vi "WT CONFIG.vi"(7 "WT 1600?":bool, 8 "error in (no error)":errorcluster, 10 "WT1600 Config ing 2":T1={"Wiring A (0: 1P2W)"=0, "Wiring B (0: 1P2W)"=0, "Wiring C (0: 1P2W)"=0, "V Range (12: 1000)"=12, "V Element (0: All)"=0, "A Element (0: All)"=0, "A Range (9: 5A)"=9, "A Sensor Ratio(mV/A) (10.0000) "=10.0, "Zero Cross Filter (0: OFF)"=0, "Line Filter (0: OFF)"=0, "PT Ratio (1.0000)"=1.0, "Scaling (F: OFF)"=FALSE, "CT Ratio (1.0000)"=1.0, "Scaling Factor (1.0000)"=1.0, "Filter Element (0: All)"=0, "Display Format (0: Numeric)"=0, "Normal Item Amount (1: 4)"=1, "Harmonics Item Amount (1: 4)"=1, "Average Type (0: OFF)"=0, "Average Count (2: 8)"=2, "A Range (9: 5A) 2"=9, "A Sensor Ratio(mV/A) (10.0000)  2"=10.0, "Zero Cross Filter (0: OFF) 2"=0, "Line Filter (0: OFF) 2"=0, "PT Ratio (1.0000) 2"=1.0, "Scaling (F: OFF) 2"=FALSE, "CT Ratio (1.0000) 2"=1.0, "Scaling Factor (1.0000) 2"=1.0, "CUT OFF FREQ"=0.0} {"Scaling Factor (1.0000) 2" min=0.0001 max=99999.9999 step=0.0001 format="%.4f"; "CT Ratio (1.0000) 2" min=0.0001 max=99999.9999 step=0.0001 format="%.4f"; "PT Ratio (1.0000) 2" min=0.0001 max=99999.9999 step=0.0001 format="%.4f"; "Line Filter (0: OFF) 2" items=["OFF", "500Hz", "5.5kHz"]; "Zero Cross Filter (0: OFF) 2" items=["OFF", "500Hz"]; "A Sensor Ratio(mV/A) (10.0000)  2" min=0.0001 max=99999.9999 step=0.0001 format="%.4f"; "A Range (9: 5A) 2" items=["AUTO", "10 mA", "20 mA", "50 mA", "100 mA", "200 mA", "500 mA", "1 A", "2 A", "5 A", "10 A", "20 A", "50 A", "S-AUTO", "50 mV", "100 mV", "250 mV", "500 mV", "1 V", "2.5 V", "5 V", "10 V"]; "Average Count (2: 8)" items=["2", "4", "8", "16", "32", "64", "128", "256"]; "Average Type (0: OFF)" items=["OFF", "Linear", "Exponent"]; "Harmonics Item Amount (1: 4)" items=["-", "4", "8", "16", "Single List", "Dual List", "Sigma List"]; "Normal Item Amount (1: 4)" items=["ALL", "4", "8", "16", "42", "78"]; "Display Format (0: Numeric)" items=["Numeric", "Wave", "Bar", "Vector", "Trend", "Numeric & Wave", "Numeric & Bar", "Numeric & Trend", "Wave & Bar", "Wave & Trend", "Bar & Trend", "Information"]; "Filter Element (0: All)" items=["All", "Element 1", "Element 2", "Element 3", "Element 4", "Element 5", "Element 6"]; "Scaling Factor (1.0000)" min=0.0001 max=99999.9999 step=0.0001 format="%.4f"; "CT Ratio (1.0000)" min=0.0001 max=99999.9999 step=0.0001 format="%.4f"; "PT Ratio (1.0000)" min=0.0001 max=99999.9999 step=0.0001 format="%.4f"; "Line Filter (0: OFF)" items=["OFF", "500Hz", "5.5kHz"]; "Zero Cross Filter (0: OFF)" items=["OFF", "500Hz"]; "A Sensor Ratio(mV/A) (10.0000)" min=0.0001 max=99999.9999 step=0.0001 format="%.4f"; "A Range (9: 5A)" items=["AUTO", "10 mA", "20 mA", "50 mA", "100 mA", "200 mA", "500 mA", "1 A", "2 A", "5 A", "10 A", "20 A", "50 A", "S-AUTO", "50 mV", "100 mV", "250 mV", "500 mV", "1 V", "2.5 V", "5 V", "10 V"]; "A Element (0: All)" items=["All", "Element 1", "Element 2", "Element 3", "Element 4", "Element 5", "Element 6"]; "V Element (0: All)" items=["All", "Element 1", "Element 2", "Element 3", "Element 4", "Element 5", "Element 6"]; "V Range (12: 1000)" items=["AUTO", "1.5", "3", "6", "10", "15", "30", "60", "100", "150", "300", "600", "1000"]; "Wiring C (0: 1P2W)" items=["1P2W", "1P3W", "3P3W", "3P4W", "3V3A", "NONE"]; "Wiring B (0: 1P2W)" items=["1P2W", "1P3W", "3P3W", "3P4W", "3V3A", "NONE"]; "Wiring A (0: 1P2W)" items=["1P2W", "1P3W", "3P3W", "3P4W", "3V3A"]}, 11 "VISA Refnum in":refnum<visa-resource-name>) -> (0 "error OUT":errorcluster, 3 "VISA OUT":refnum<visa-resource-name>)   [LabVIEW 2019]
panel:
  # "ON\nOFF"
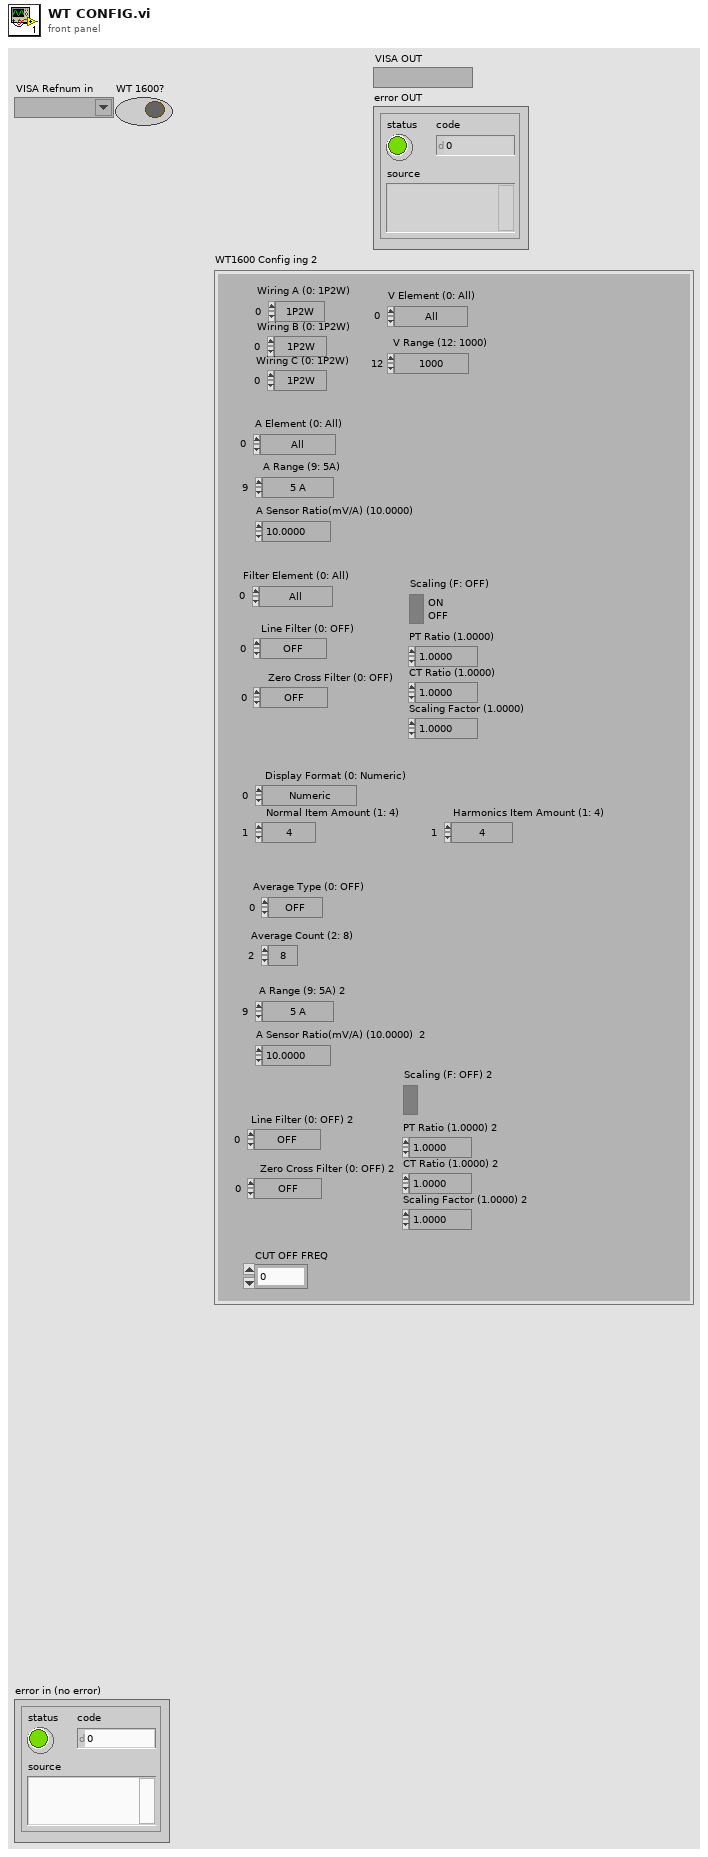
[diagram p1: front panel]
types:
  T1 = cluster{"Wiring A (0: 1P2W)":u16, "Wiring B (0: 1P2W)":u16, "Wiring C (0: 1P2W)":u16, "V Range (12: 1000)":u16, "V Element (0: All)":u16, "A Element (0: All)":u16, "A Range (9: 5A)":u16, "A Sensor Ratio(mV/A) (10.0000) ":dbl, "Zero Cross Filter (0: OFF)":u16, "Line Filter (0: OFF)":u16, "PT Ratio (1.0000)":dbl, "Scaling (F: OFF)":bool, "CT Ratio (1.0000)":dbl, "Scaling Factor (1.0000)":dbl, "Filter Element (0: All)":u16, "Display Format (0: Numeric)":u16, "Normal Item Amount (1: 4)":u16, "Harmonics Item Amount (1: 4)":u16, "Average Type (0: OFF)":u16, "Average Count (2: 8)":u16, "A Range (9: 5A) 2":u16, "A Sensor Ratio(mV/A) (10.0000)  2":dbl, "Zero Cross Filter (0: OFF) 2":u16, "Line Filter (0: OFF) 2":u16, "PT Ratio (1.0000) 2":dbl, "Scaling (F: OFF) 2":bool, "CT Ratio (1.0000) 2":dbl, "Scaling Factor (1.0000) 2":dbl, "CUT OFF FREQ":dbl}
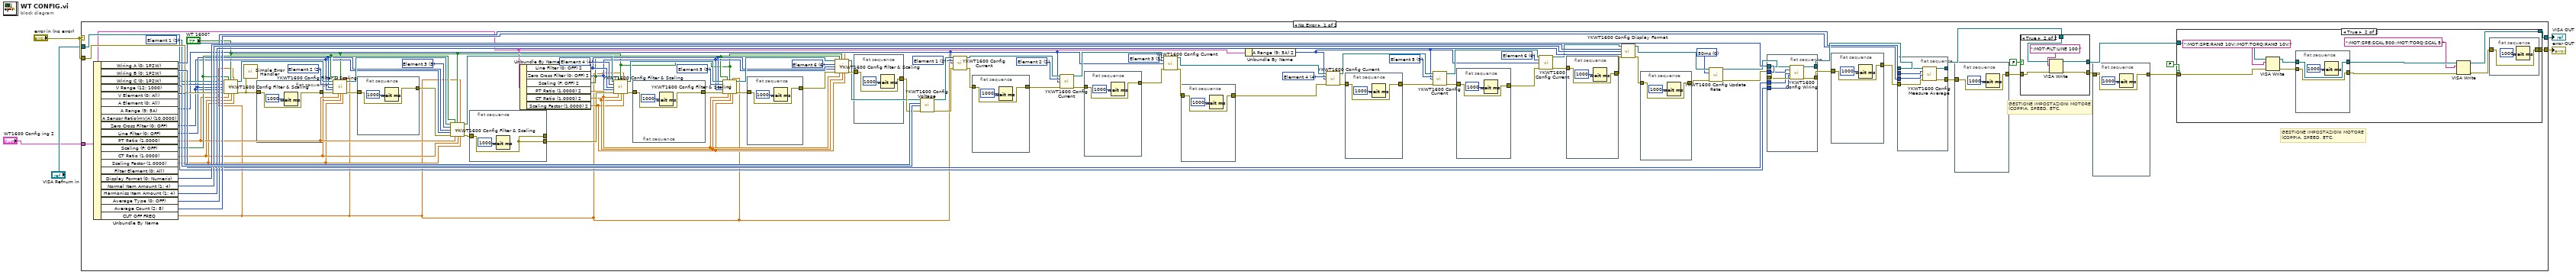
[diagram p0: block diagram]
diagram:
  n1 = case shown="No Error" "error in (no error)" {
    tunnel: "WT1600 Config ing 2" -> [w13 _]
    tunnel: "error in (no error)" -> [w76 w175]
    tunnel: "VISA Refnum in" -> [w75 w174]
    tunnel: [w74 w174] -> w3
    tunnel: [w73 w175] -> w2
    frame No Error {
      w26 = u16 6 items=["All", "Element 1", "Element 2", "Element 3", "Element 4", "Element 5", "Element 6"] ("Element (0: All)")
      w25 = u16 5 items=["All", "Element 1", "Element 2", "Element 3", "Element 4", "Element 5", "Element 6"] ("Element (0: All)")
      w24 = u16 4 items=["All", "Element 1", "Element 2", "Element 3", "Element 4", "Element 5", "Element 6"] ("Element (0: All)")
      w22 = u16 3 items=["All", "Element 1", "Element 2", "Element 3", "Element 4", "Element 5", "Element 6"] ("Element (0: All)")
      w23 = u16 2 items=["All", "Element 1", "Element 2", "Element 3", "Element 4", "Element 5", "Element 6"] ("Element (0: All)")
      w21 = u16 1 items=["All", "Element 1", "Element 2", "Element 3", "Element 4", "Element 5", "Element 6"] ("Element (0: All)")
      w52 = u16 6 items=["All", "Element 1", "Element 2", "Element 3", "Element 4", "Element 5", "Element 6"] ("Element (0: All)")
      w53 = u16 5 items=["All", "Element 1", "Element 2", "Element 3", "Element 4", "Element 5", "Element 6"] ("Element (0: All)")
      w54 = u16 4 items=["All", "Element 1", "Element 2", "Element 3", "Element 4", "Element 5", "Element 6"] ("Element (0: All)")
      w55 = u16 3 items=["All", "Element 1", "Element 2", "Element 3", "Element 4", "Element 5", "Element 6"] ("Element (0: All)")
      w51 = u16 2 items=["All", "Element 1", "Element 2", "Element 3", "Element 4", "Element 5", "Element 6"] ("Element (0: All)")
      w56 = u16 1 items=["All", "Element 1", "Element 2", "Element 3", "Element 4", "Element 5", "Element 6"] ("Element (0: All)")
      w82 = u16 0 items=["50ms", "100ms", "200ms", "500ms", "1s", "2s", "5s"] ("Update Rate (3: 500ms)")
      # "GESTIONE IMPOSTAZIONI MOTORE\n(COPPIA, SPEED, ETC."
      # "GESTIONE IMPOSTAZIONI MOTORE\n(COPPIA, SPEED, ETC."
      n2 = Unbundle By Name(w13) -> ("Wiring A (0: 1P2W)"=w93:u16, "Wiring B (0: 1P2W)"=w92:u16, "Wiring C (0: 1P2W)"=w91:u16, "V Range (12: 1000)"=w101:u16, "V Element (0: All)"=w100:u16, "A Range (9: 5A)"=w20:u16, "Zero Cross Filter (0: OFF)"=w48:u16, "Line Filter (0: OFF)"=w49:u16, "PT Ratio (1.0000)"=w47:dbl, "Scaling (F: OFF)"=w50:bool, "CT Ratio (1.0000)"=w46:dbl, "Scaling Factor (1.0000)"=w45:dbl, "Display Format (0: Numeric)"=w99:u16, "Normal Item Amount (1: 4)"=w98:u16, "Harmonics Item Amount (1: 4)"=w97:u16, "Average Type (0: OFF)"=w95:u16, "Average Count (2: 8)"=w94:u16, "CUT OFF FREQ"=w6:dbl)  [unwired: 3 out]
      n3 = call "YKWT1600 Config Filter & Scaling.vi"("VISA session"=w75, "Scaling (F: OFF)"=w50, "WT 1600?"="WT 1600?", "Cutoff Frequency (0.5 kHz)"=w6, "Element (0: All)"=w56, "Line Filter (0: OFF)"=w49, "WT 1600 Zero Cross Filter (0: OFF)"=w48, "error in (no error)"=w76, "PT Ratio (1.0000)"=w47, "CT Ratio (1.0000)"=w46, "Scaling Factor (1.0000)"=w45) -> ("dup VISA session"=w72:refnum<visa-resource-name>, "error out"=w10:errorcluster)  [unwired: 3 out]
      n4 = call <vilib>:"Simple Error Handler.vi"("error in (no error)"=w10) -> ()  [unwired: 4 in, 5 out]
      n5 = flat-sequence {
        tunnel: w10 -> [w165]
        tunnel: [w165] -> w9
        frame #0 {
          n6 = Wait (ms)(milliseconds to wait=1000) -> ()  [unwired: 1 out]
        }
      }
      n7 = call "YKWT1600 Config Filter & Scaling.vi"("VISA session"=w72, "Scaling (F: OFF)"=w50, "WT 1600?"="WT 1600?", "Cutoff Frequency (0.5 kHz)"=w6, "Element (0: All)"=w51, "Line Filter (0: OFF)"=w49, "WT 1600 Zero Cross Filter (0: OFF)"=w48, "error in (no error)"=w9, "PT Ratio (1.0000)"=w47, "CT Ratio (1.0000)"=w46, "Scaling Factor (1.0000)"=w45) -> ("dup VISA session"=w58:refnum<visa-resource-name>, "error out"=w71:errorcluster)  [unwired: 3 out]
      n8 = flat-sequence {
        tunnel: w71 -> [w163]
        tunnel: [w163] -> w70
        frame #0 {
          n9 = Wait (ms)(milliseconds to wait=1000) -> ()  [unwired: 1 out]
        }
      }
      n10 = call "YKWT1600 Config Filter & Scaling.vi"("VISA session"=w58, "Scaling (F: OFF)"=w50, "WT 1600?"="WT 1600?", "Cutoff Frequency (0.5 kHz)"=w6, "Element (0: All)"=w55, "Line Filter (0: OFF)"=w49, "WT 1600 Zero Cross Filter (0: OFF)"=w48, "error in (no error)"=w70, "PT Ratio (1.0000)"=w47, "CT Ratio (1.0000)"=w46, "Scaling Factor (1.0000)"=w45) -> ("dup VISA session"=w61:refnum<visa-resource-name>, "error out"=w69:errorcluster)  [unwired: 3 out]
      n11 = flat-sequence {
        tunnel: [w160] -> _
        tunnel: [w160] -> w68
        tunnel: w69 -> [w160]
        frame #0 {
          n12 = Wait (ms)(milliseconds to wait=1000) -> ()  [unwired: 1 out]
        }
      }
      n13 = Unbundle By Name(w13) -> ("Line Filter (0: OFF) 2"=w19:u16, "Zero Cross Filter (0: OFF) 2"=w18:u16, "Scaling (F: OFF) 2"=w17:bool, "PT Ratio (1.0000) 2"=w16:dbl, "CT Ratio (1.0000) 2"=w15:dbl, "Scaling Factor (1.0000) 2"=w14:dbl)
      n14 = call "YKWT1600 Config Filter & Scaling.vi"("VISA session"=w61, "Scaling (F: OFF)"=w17, "WT 1600?"="WT 1600?", "Cutoff Frequency (0.5 kHz)"=w6, "Element (0: All)"=w54, "Line Filter (0: OFF)"=w19, "WT 1600 Zero Cross Filter (0: OFF)"=w18, "error in (no error)"=w68, "PT Ratio (1.0000)"=w16, "CT Ratio (1.0000)"=w15, "Scaling Factor (1.0000)"=w14) -> ("dup VISA session"=w60:refnum<visa-resource-name>, "error out"=w67:errorcluster)  [unwired: 3 out]
      n15 = flat-sequence {
        tunnel: w67 -> [w159]
        tunnel: [w159] -> w66
        frame #0 {
          n16 = Wait (ms)(milliseconds to wait=1000) -> ()  [unwired: 1 out]
        }
      }
      n17 = call "YKWT1600 Config Filter & Scaling.vi"("VISA session"=w60, "Scaling (F: OFF)"=w17, "WT 1600?"="WT 1600?", "Cutoff Frequency (0.5 kHz)"=w6, "Element (0: All)"=w53, "Line Filter (0: OFF)"=w19, "WT 1600 Zero Cross Filter (0: OFF)"=w18, "error in (no error)"=w66, "PT Ratio (1.0000)"=w16, "CT Ratio (1.0000)"=w15, "Scaling Factor (1.0000)"=w14) -> ("dup VISA session"=w59:refnum<visa-resource-name>, "error out"=w65:errorcluster)  [unwired: 3 out]
      n18 = flat-sequence {
        tunnel: w65 -> [w157]
        tunnel: [w157] -> w64
        frame #0 {
          n19 = Wait (ms)(milliseconds to wait=1000) -> ()  [unwired: 1 out]
        }
      }
      n20 = call "YKWT1600 Config Filter & Scaling.vi"("VISA session"=w59, "Scaling (F: OFF)"=w17, "WT 1600?"="WT 1600?", "Cutoff Frequency (0.5 kHz)"=w6, "Element (0: All)"=w52, "Line Filter (0: OFF)"=w19, "WT 1600 Zero Cross Filter (0: OFF)"=w18, "error in (no error)"=w64, "PT Ratio (1.0000)"=w16, "CT Ratio (1.0000)"=w15, "Scaling Factor (1.0000)"=w14) -> ("dup VISA session"=w57:refnum<visa-resource-name>, "error out"=w63:errorcluster)  [unwired: 3 out]
      n21 = flat-sequence {
        tunnel: w63 -> [w155]
        tunnel: [w155] -> w62
        frame #0 {
          n22 = Wait (ms)(milliseconds to wait=1000) -> ()  [unwired: 1 out]
        }
      }
      n23 = call "YKWT1600 Config Voltage.vi"("VISA session"=w57, "Element (0: All)"=w100, "V Range (12: 1000)"=w101, "error in (no error)"=w62) -> ("dup VISA session"=w103:refnum<visa-resource-name>, "error out"=w102:errorcluster)  [unwired: 10 out]
      n24 = call "YKWT1600 Config Current.vi"("VISA session"=w103, "Element (0: All)"=w21, "A Range (9: 5A)"=w20, "error in (no error)"=w102) -> ("dup VISA session"=w28:refnum<visa-resource-name>, "error out"=w34:errorcluster)  [unwired: 1 in, 9 out]
      n25 = flat-sequence {
        tunnel: w34 -> [w153]
        tunnel: [w153] -> w44
        frame #0 {
          n26 = Wait (ms)(milliseconds to wait=1000) -> ()  [unwired: 1 out]
        }
      }
      n27 = call "YKWT1600 Config Current.vi"("VISA session"=w28, "Element (0: All)"=w23, "A Range (9: 5A)"=w20, "error in (no error)"=w44) -> ("dup VISA session"=w32:refnum<visa-resource-name>, "error out"=w43:errorcluster)  [unwired: 1 in, 9 out]
      n28 = flat-sequence {
        tunnel: w43 -> [w151]
        tunnel: [w151] -> w42
        frame #0 {
          n29 = Wait (ms)(milliseconds to wait=1000) -> ()  [unwired: 1 out]
        }
      }
      n30 = call "YKWT1600 Config Current.vi"("VISA session"=w32, "Element (0: All)"=w22, "A Range (9: 5A)"=w20, "error in (no error)"=w42) -> ("dup VISA session"=w31:refnum<visa-resource-name>, "error out"=w41:errorcluster)  [unwired: 1 in, 9 out]
      n31 = flat-sequence {
        tunnel: w41 -> [w149]
        tunnel: [w149] -> w40
        frame #0 {
          n32 = Wait (ms)(milliseconds to wait=1000) -> ()  [unwired: 1 out]
        }
      }
      n33 = Unbundle By Name(w13) -> ("A Range (9: 5A) 2"=w12:u16)
      n34 = call "YKWT1600 Config Current.vi"("VISA session"=w31, "Element (0: All)"=w24, "A Range (9: 5A)"=w12, "error in (no error)"=w40) -> ("dup VISA session"=w30:refnum<visa-resource-name>, "error out"=w39:errorcluster)  [unwired: 1 in, 9 out]
      n35 = flat-sequence {
        tunnel: w39 -> [w147]
        tunnel: [w147] -> w38
        frame #0 {
          n36 = Wait (ms)(milliseconds to wait=1000) -> ()  [unwired: 1 out]
        }
      }
      n37 = call "YKWT1600 Config Current.vi"("VISA session"=w30, "Element (0: All)"=w25, "A Range (9: 5A)"=w12, "error in (no error)"=w38) -> ("dup VISA session"=w29:refnum<visa-resource-name>, "error out"=w37:errorcluster)  [unwired: 1 in, 9 out]
      n38 = flat-sequence {
        tunnel: [w144] -> w36
        tunnel: w37 -> [w144]
        frame #0 {
          n39 = Wait (ms)(milliseconds to wait=1000) -> ()  [unwired: 1 out]
        }
      }
      n40 = call "YKWT1600 Config Current.vi"("VISA session"=w29, "Element (0: All)"=w26, "A Range (9: 5A)"=w12, "error in (no error)"=w36) -> ("dup VISA session"=w27:refnum<visa-resource-name>, "error out"=w35:errorcluster)  [unwired: 1 in, 9 out]
      n41 = flat-sequence {
        tunnel: [w142] -> w33
        tunnel: w35 -> [w142]
        frame #0 {
          n42 = Wait (ms)(milliseconds to wait=1000) -> ()  [unwired: 1 out]
        }
      }
      n43 = call "YKWT1600 Config Display Format.vi"("VISA session"=w27, "Display Format (0: Numeric)"=w99, "Normal Item Amount (1: 4)"=w98, "Harmonics Item Amount (1: 4)"=w97, "error in (no error)"=w33) -> ("dup VISA session"=w86:refnum<visa-resource-name>, "error out"=w87:errorcluster)  [unwired: 9 out]
      n44 = flat-sequence {
        tunnel: w87 -> [w171]
        tunnel: [w171] -> w84
        frame #0 {
          n45 = Wait (ms)(milliseconds to wait=1000) -> ()  [unwired: 1 out]
        }
      }
      n46 = call "YKWT1600 Config Update Rate.vi"("VISA session"=w86, "Update Rate (3: 500ms)"=w82, "error in (no error)"=w84) -> ("dup VISA session"=w85:refnum<visa-resource-name>, "error out"=w83:errorcluster)  [unwired: 11 in]
      n47 = flat-sequence {
        tunnel: [w134] -> w96
        tunnel: [w135] -> w78
        tunnel: w85 -> [w133]
        tunnel: w83 -> [w132]
        tunnel: w91 -> [w129]
        tunnel: w92 -> [w130]
        tunnel: w93 -> [w131]
        frame #0 {
          n48 = call "YKWT1600 Config Wiring.vi"("VISA session"=w133, "Wiring A (0: 1P2W)"=w131, "Wiring B (0: 1P2W)"=w130, "Wiring C (0: 1P2W)"=w129, "error in (no error)"=w132) -> ("dup VISA session"=w134:refnum<visa-resource-name>, "error out"=w135:errorcluster)  [unwired: 9 out]
        }
      }
      n49 = flat-sequence {
        tunnel: w78 -> [w166]
        tunnel: [w166] -> w77
        frame #0 {
          n50 = Wait (ms)(milliseconds to wait=1000) -> ()  [unwired: 1 out]
        }
      }
      n51 = flat-sequence {
        tunnel: w96 -> [w141]
        tunnel: [w140] -> w90
        tunnel: w77 -> [w139]
        tunnel: [w138] -> w80
        tunnel: w95 -> [w137]
        tunnel: w94 -> [w136]
        frame #0 {
          n52 = call "YKWT1600 Config Measure Average.vi"("VISA session"=w141, "Average Type (0: OFF)"=w137, "Average Count (2: 8)"=w136, "error in (no error)"=w139) -> ("dup VISA session"=w140:refnum<visa-resource-name>, "error out"=w138:errorcluster)  [unwired: 10 out]
        }
      }
      n53 = flat-sequence {
        tunnel: w80 -> [w169]
        tunnel: [w169] -> w79
        frame #0 {
          n54 = Wait (ms)(milliseconds to wait=1000) -> ()  [unwired: 1 out]
        }
      }
      n55 = case shown="True" FALSE {
        tunnel: w90 -> [w104 w109]
        tunnel: [w105 w106] -> w89
        tunnel: [w104 w107] -> w81
        tunnel: w79 -> [w105 w108]
        frame False {
        }
        frame True {
          n56 = VISA Write(VISA resource name=w109, write buffer=":MOT:FILT:LINE 100;", error in (no error)=w108) -> (VISA resource name out=w107:refnum<visa-resource-name>, error out=w106:errorcluster)  [unwired: 1 out]
        }
      }
      n57 = flat-sequence {
        tunnel: w89 -> [w173]
        tunnel: [w173] -> w88
        frame #0 {
          n58 = Wait (ms)(milliseconds to wait=1000) -> ()  [unwired: 1 out]
        }
      }
      n59 = case shown="True" FALSE {
        tunnel: w88 -> [w111 w122]
        tunnel: w81 -> [w112 w120]
        tunnel: [w112 w115] -> w74
        tunnel: [w111 w123] -> w73
        frame False {
        }
        frame True {
          n60 = VISA Write(VISA resource name=w120, write buffer=":MOT:SPE:RANG 10V;:MOT:TORQ:RANG 10V;", error in (no error)=w122) -> (VISA resource name out=w119:refnum<visa-resource-name>, error out=w113:errorcluster)  [unwired: 1 out]
          n61 = flat-sequence {
            tunnel: w113 -> [w127]
            tunnel: [w127] -> w114
            tunnel: w119 -> [w128]
            tunnel: [w128] -> w118
            frame #0 {
              n62 = Wait (ms)(milliseconds to wait=1000) -> ()  [unwired: 1 out]
            }
          }
          n63 = VISA Write(VISA resource name=w118, write buffer=":MOT:SPE:SCAL 500;:MOT:TORQ:SCAL 5;", error in (no error)=w114) -> (VISA resource name out=w115:refnum<visa-resource-name>, error out=w116:errorcluster)  [unwired: 1 out]
          n64 = flat-sequence {
            tunnel: w116 -> [w125]
            tunnel: [w125] -> w123
            frame #0 {
              n65 = Wait (ms)(milliseconds to wait=1000) -> ()  [unwired: 1 out]
            }
          }
        }
      }
    }
    frame Error {
    }
  }
  "VISA OUT" <- w3
  "error OUT" <- w2
